vi "Mask.vi"(0 "Image In":T2, 1 "ROI Descriptor (Image Mask 1)":T1 {"Contours"."Type" items=["No Selection", "Point", "Line", "Rectangle", "Oval", "Polygon", "Freehand Region", "Annulus", "Unused2", "Unused3", "Broken Line", "Freehand Line", "Rotated Rectangle"]}, 7 "error in":errorcluster) -> (20 "Image Out":T2, 27 "error out":errorcluster)   [LabVIEW 2009]
uses:
  <vilib>/vision/Image Controls.llb/IMAQ Image.ctl
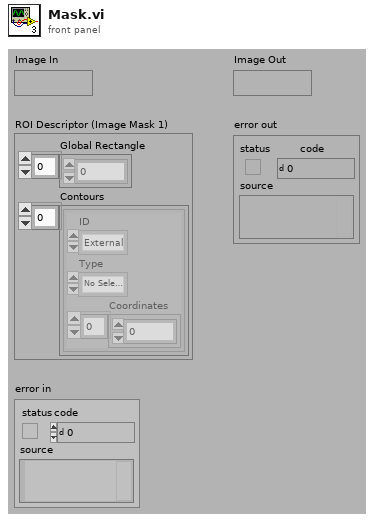
[diagram p1: front panel]
types:
  T1 = cluster{"Global Rectangle":i32[], "Contours":cluster{"ID":enum32{"External", "Internal"}, "Type":u32, "Coordinates":i32[]}[]}
  T2 = typedef "IMAQ Image.ctl" = refnum<image>
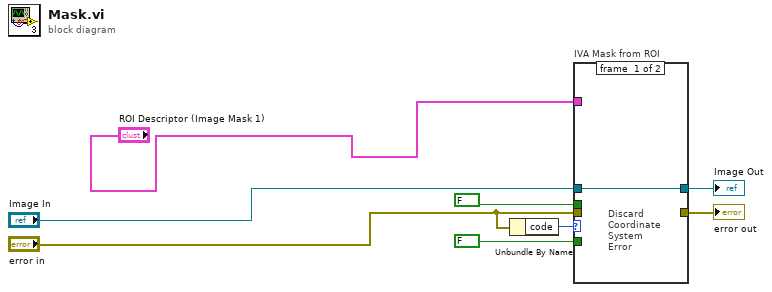
[diagram p0: block diagram]
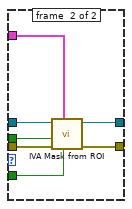
[diagram p2: hidden frame]
diagram:
  n1 = Unbundle By Name("error in") -> ("code"=w1:i32)
  n2 = case "IVA Mask from ROI" shown="Default" w1 {
    tunnel: "ROI Descriptor (Image Mask 1)" -> [_ w16]
    tunnel: FALSE ("Shrink") -> [_ w15]
    tunnel: "Image In" -> [w9 w14]
    tunnel: "error in" -> [_ w13]
    tunnel: [_ w12] -> w4
    tunnel: [w9 w11] -> w3
    tunnel: FALSE ("Out / In") -> [_ w10]
    frame #0 {
      # "Discard\nCoordinate\nSystem\nError"
    }
    frame #1 {
      n3 = call <vilib>:"IVA Mask from ROI.vi"("Shrink"=w15, "ROI Descriptor"=w16, "error in (no error)"=w13, "Out / In"=w10, "Image Src"=w14) -> ("error out"=w12:errorcluster, "Image Out"=w11:T2)  [unwired: 5 out]
    }
  }
  "error out" <- w4
  "Image Out" <- w3
